vi "关键参数交互.vi"(9 "量程下拉列表":refnum<vi>, 10 "测量模式下拉列表":refnum<vi>, 11 "参数下拉列表":refnum<vi>) -> ()   [LabVIEW 2016]
uses:
  <vilib>/regexp/Match Regular Expression.xnode
panel:
  out "x != y?":T1
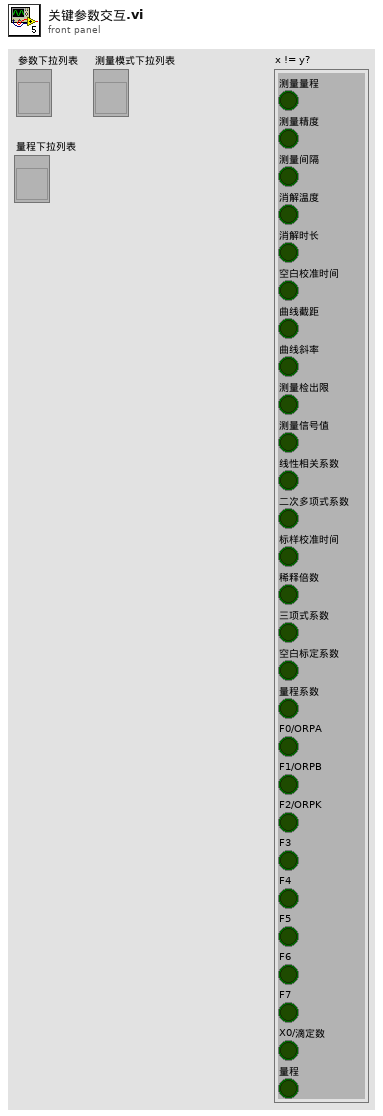
[diagram p1: front panel]
types:
  T1 = cluster{"测量量程":bool, "测量精度":bool, "测量间隔":bool, "消解温度":bool, "消解时长":bool, "空白校准时间":bool, "曲线截距":bool, "曲线斜率":bool, "测量检出限":bool, "测量信号值":bool, "线性相关系数":bool, "二次多项式系数":bool, "标样校准时间":bool, "稀释倍数":bool, "三项式系数":bool, "空白标定系数":bool, "量程系数":bool, "F0/ORPA":bool, "F1/ORPB":bool, "F2/ORPK":bool, "F3":bool, "F4":bool, "F5":bool, "F6":bool, "F7":bool, "X0/滴定数":bool, "量程":bool}
  T2 = cluster{"chose":string, "公式":cluster{"X^2":dbl, "X":dbl, "b":dbl}}
  T3 = cluster{"测量量程":dbl, "测量精度":dbl, "测量间隔":dbl, "消解温度":dbl, "消解时长":dbl, "空白校准时间":timestamp, "曲线截距":dbl, "曲线斜率":dbl, "测量检出限":dbl, "测量信号值":dbl, "线性相关系数":dbl, "二次多项式系数":dbl, "标样校准时间":timestamp, "稀释倍数":dbl, "三项式系数":dbl, "空白标定系数":dbl, "量程系数":dbl, "F0/ORPA":dbl, "F1/ORPB":dbl, "F2/ORPK":dbl, "F3":dbl, "F4":dbl, "F5":dbl, "F6":dbl, "F7":dbl, "X0/滴定数":dbl, "量程":dbl}
  T4 = cluster{"时间标识":timestamp, "设备":string, "日志信息":string, "流程参数":string}
  T5 = enum16{"", "水样测量", "标样核查", "零点核查", "跨度核查", "空白测试", "平行样测试", "加标回收"}
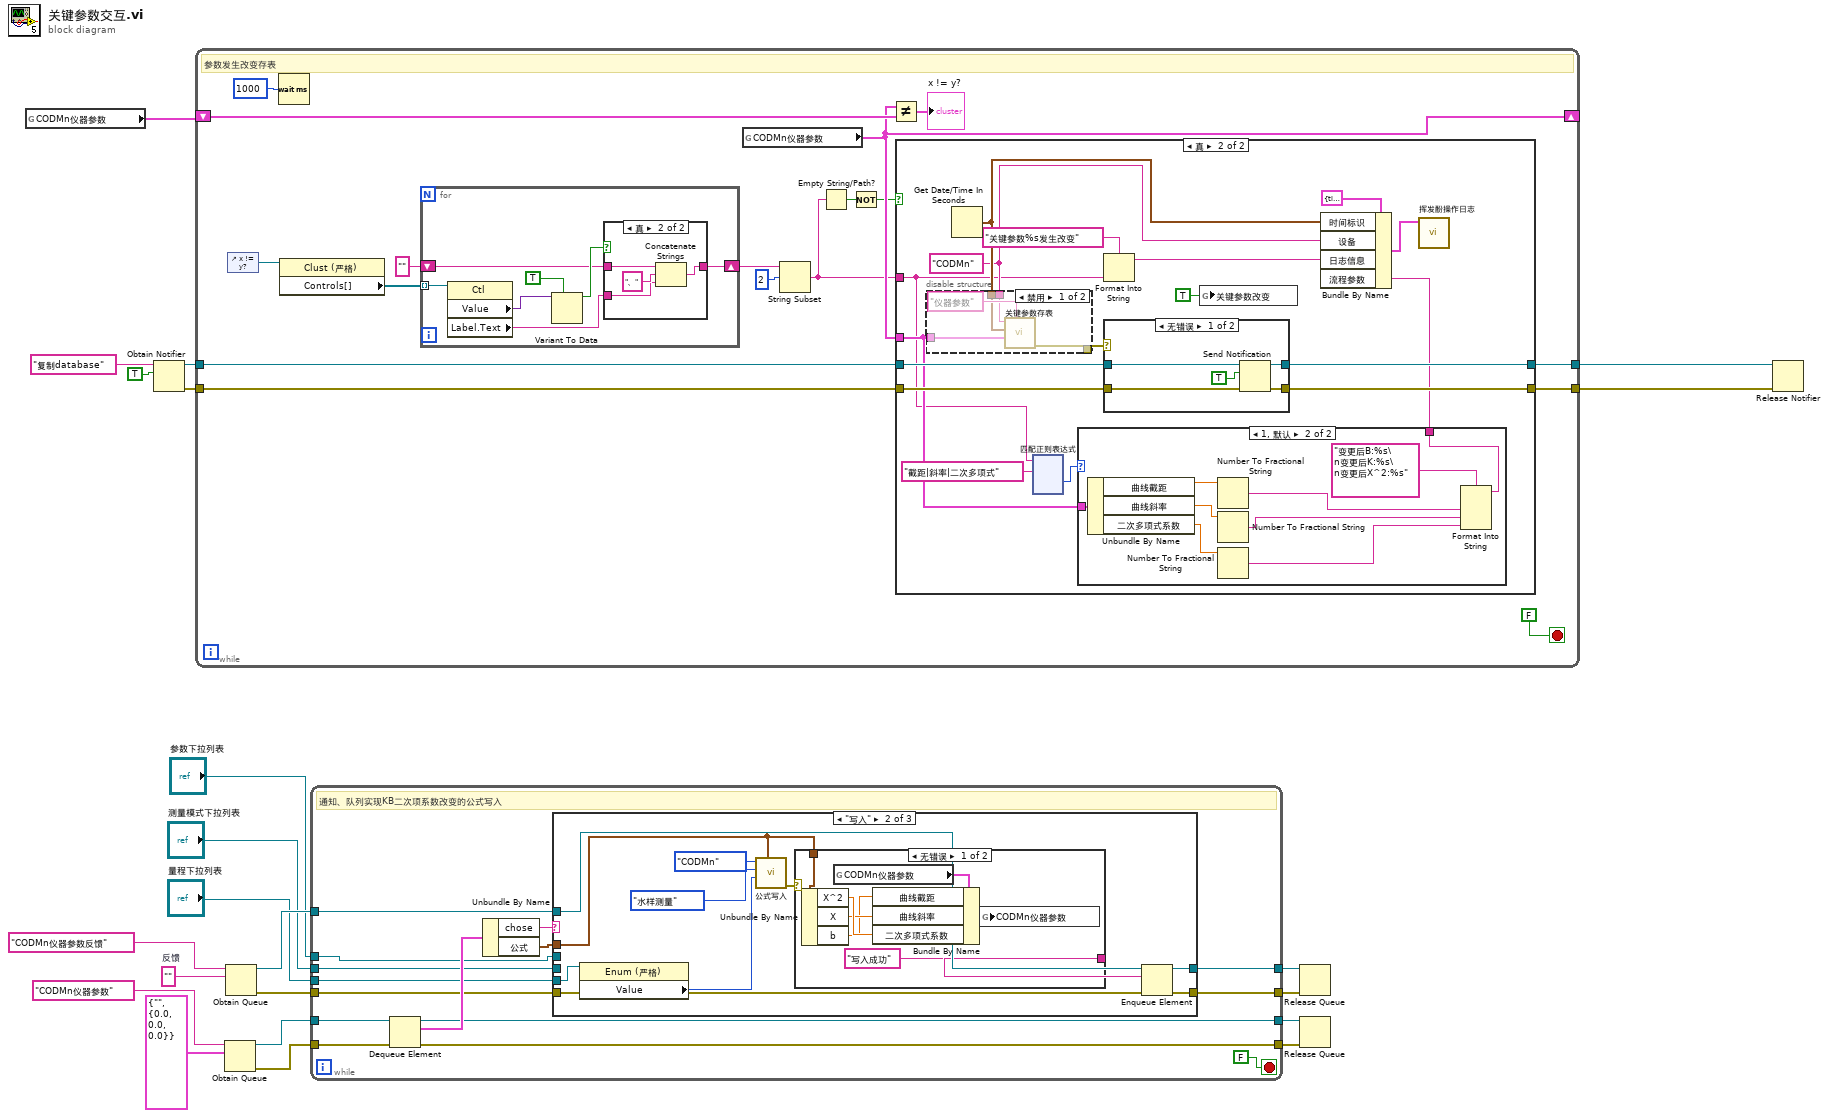
[diagram p0: block diagram]
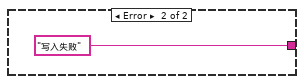
[diagram p3: hidden frame]
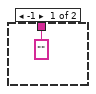
[diagram p8: hidden frame]
diagram:
  w15 = ""  # 反馈
  n1 = global read "挥发酚断电保存全局变量.vi" "CODMn仪器参数"() -> (w22:T3)
  n2 = Obtain Notifier(name (unnamed)="复制database" ("名称（未命名）"), notification data type=TRUE) -> (notifier out=w5:refnum<notifier>, error out=w4:errorcluster)  [unwired: 2 in, 1 out]
  n3 = while {
    shift-right: [w34] -> _
    shift-left: w22 -> [w37]
    tunnel: w5 -> [w33]
    tunnel: w4 -> [w32]
    tunnel: [w31] -> w3
    tunnel: [w30] -> w2
    stop <- FALSE stop-if-true
    # "参数发生改变存表"
    n4 = control-ref of="x != y?"() -> (w35:refnum<vi>)
    n5 = Wait (ms)(milliseconds to wait=u32 1000 ("等待时间（毫秒）")) -> ()  [unwired: 1 out]
    n6 = property class="Clust (严格)"(reference=w35) -> ("Controls[]"=w26:refnum<vi>[])  [unwired: 1 in, 2 out]
    n7 = for {
      tunnel: w26 -> [w46] mode=indexing
      shift-right: [w40] -> w28
      shift-left: "" -> [w42]
      n8 = property class="Ctl"(reference=w46) -> ("Value"=w44:variant, "Label.Text"=w41:string)  [unwired: 1 in, 2 out]
      n9 = Variant To Data(type=TRUE, Variant=w44) -> (data=w43:bool)  [unwired: 1 in, 1 out]
      n10 = case shown="真" w43 {
        tunnel: w42 -> [w47 w51]
        tunnel: w41 -> [_ w48]
        tunnel: [w47 w50] -> w40
        frame False {
        }
        frame True {
          n11 = Concatenate Strings(w51, "、", w48) -> (w50:string)
        }
      }
    }
    n12 = global read "挥发酚断电保存全局变量.vi" "CODMn仪器参数"() -> (w34:T3)
    n13 = String Subset(string=w28, offset (0)=2 ("偏移量(0)")) -> (substring=w23:string)  [unwired: 1 in]
    n14 = Empty String/Path?(string/path=w23) -> (empty?=w25:bool)
    n15 = Not(x=w25) -> (.not. x?=w24:bool)
    n16 = Not Equal?(x=w34, y=w37) -> (x != y?=→"x != y?":T1)
    n17 = case shown="真" w24 {
      tunnel: w34 -> [_ w59]
      tunnel: w23 -> [_ w56]
      tunnel: w33 -> [w53 w64]
      tunnel: w32 -> [w52 w63]
      tunnel: [w53 w61] -> w31
      tunnel: [w52 w60] -> w30
      frame False {
      }
      frame True {
        w67 = "CODMn" ("仪器名称")
        n18 = Get Date/Time In Seconds() -> (seconds since 1Jan1904=w68:timestamp)
        n19 = disable-structure shown="禁用" {
          disable-tunnel: w68 -> [w74 _]
          disable-tunnel: w67 -> [w73 _]
          disable-tunnel: [w72 _] -> w62
          disable-tunnel: w59 -> [w71 _]
          frame Disabled {
            n20 = call "关键参数存表.vi"("table"="仪器参数", "仪器参数"=w71, "datatime"=w74, "仪器名称"=w73) -> ("error out"=w72:errorcluster)  [unwired: 7 in]
          }
          frame Enabled {
          }
        }
        n21 = xnode "匹配正则表达式"("输入字符串"=w56, "正则表达式"="截距|斜率|二次多项式") -> ("匹配后偏移量"=w55:i32)  [unwired: 4 in, 4 out]
        n22 = case shown="1, 默认" w55 {
          tunnel: w59 -> [_ w198]
          tunnel: ["" w191] -> w58
          frame -1 {
          }
          frame 1, Default {
            n23 = Unbundle By Name(w198) -> ("曲线截距"=w197:dbl, "曲线斜率"=w196:dbl, "二次多项式系数"=w195:dbl)
            n24 = Number To Fractional String(number=w197) -> (F-format string=w194:string)  [unwired: 3 in]
            n25 = Number To Fractional String(number=w196) -> (F-format string=w193:string)  [unwired: 3 in]
            n26 = Number To Fractional String(number=w195) -> (F-format string=w192:string)  [unwired: 3 in]
            n27 = Format Into String(format string="变更后B:%s\n变更后K:%s\n变更后X^2:%s" ("格式字符串"), w194, w193, w192) -> (resulting string=w191:string)  [unwired: 2 in, 1 out]
          }
        }
        n28 = Format Into String(format string="关键参数%s发生改变" ("格式字符串"), w56) -> (resulting string=w65:string)  [unwired: 2 in, 1 out]
        n29 = case shown="无错误" w62 {
          tunnel: w64 -> [w204 w206]
          tunnel: w63 -> [w203 w205]
          tunnel: [w201 w206] -> w61
          tunnel: [w200 w205] -> w60
          frame No Error {
            n30 = Send Notification(notification=TRUE ("通知"), notifier=w204, error in (no error)=w203) -> (notifier out=w201:refnum<notifier>, error out=w200:errorcluster)
          }
          frame Error {
          }
        }
        n31 = global write "挥发酚断电保存全局变量.vi" "关键参数改变"(TRUE ("关键参数改变")) -> ()
        n32 = Bundle By Name(cluster=T4 {"时间标识"=timestamp(0 s since 1904-01-01), "设备"="", "日志信息"="", "流程参数"=""} ("data in"), "时间标识"=w68, "设备"=w67, "日志信息"=w65, "流程参数"=w58) -> (w69:T4)
        n33 = call "挥发酚操作日志.vi"("data in"=w69) -> ()  [unwired: 11 in]
      }
    }
  }
  n34 = Obtain Queue(name (unnamed)="CODMn仪器参数" ("名称（未命名）"), element data type=T2 {"chose"="", "公式"={"X^2"=0.0, "X"=0.0, "b"=0.0}}) -> (queue out=w11:refnum<queue>, error out=w10:errorcluster)  [unwired: 3 in, 1 out]
  n35 = Obtain Queue(name (unnamed)="CODMn仪器参数反馈" ("名称（未命名）"), element data type=w15) -> (queue out=w16:refnum<queue>, error out=w14:errorcluster)  [unwired: 3 in, 1 out]
  n36 = while {
    tunnel: w11 -> [w220]
    tunnel: w10 -> [w219]
    tunnel: [w211] -> w19
    tunnel: [w210] -> w18
    tunnel: w16 -> [w215]
    tunnel: w14 -> [w214]
    tunnel: [w213] -> w13
    tunnel: [w212] -> w12
    tunnel: "参数下拉列表" -> [w209]
    tunnel: "测量模式下拉列表" -> [w208]
    tunnel: "量程下拉列表" -> [w207]
    stop <- FALSE stop-if-true
    # "通知、队列实现KB二次项系数改变的公式写入"
    n37 = Dequeue Element(queue=w220, error in (no error)=w219) -> (queue out=w211:refnum<queue>, element=w218:T2, error out=w210:errorcluster)  [unwired: 1 in, 1 out]
    n38 = Unbundle By Name(w218) -> ("chose"=w217:string, "公式"=w216:cluster{"X^2":dbl, "X":dbl, "b":dbl})
    n39 = case shown="\"写入\"" w217 {
      tunnel: w216 -> [_ w228 _]
      tunnel: w215 -> [w223 w233 w244]
      tunnel: w214 -> [w222 w231 w243]
      tunnel: [w223 w230 w244] -> w213
      tunnel: [w222 w229 w243] -> w212
      tunnel: w209 -> [_ _ _]
      tunnel: w208 -> [_ _ _]
      tunnel: w207 -> [_ w225 _]
      frame "假", Default {
      }
      frame "写入" {
        n40 = property class="Enum (严格)"(reference=w225) -> ("Value"=w224:enum16{"低量程1", "低量程2", "高量程1", "高量程2"})  [unwired: 1 in, 2 out]
        n41 = call "公式写入.vi"("公式"=w228, "量程"=w224, "测量模式"=T5."水样测量", "测量参数"=enum16{"CODMn"}."CODMn") -> ("error out"=w234:errorcluster)  [unwired: 7 in]
        n42 = case shown="无错误" w234 {
          tunnel: ["写入成功" ("消息") "写入失败" ("消息")] -> w232
          tunnel: w228 -> [w238 _]
          frame No Error {
            n43 = Unbundle By Name(w238) -> ("X^2"=w237:dbl, "X"=w236:dbl, "b"=w235:dbl)
            n44 = global read "挥发酚断电保存全局变量.vi" "CODMn仪器参数"() -> (w239:T3)
            n45 = Bundle By Name(cluster=w239, "曲线截距"=w235, "曲线斜率"=w236, "二次多项式系数"=w237) -> (w240:T3)
            n46 = global write "挥发酚断电保存全局变量.vi" "CODMn仪器参数"(w240) -> ()
          }
          frame Error {
          }
        }
        n47 = Enqueue Element(queue=w233, element=w232, error in (no error)=w231) -> (queue out=w230:refnum<queue>, error out=w229:errorcluster)  [unwired: 1 in, 1 out]
      }
      frame "读取" {
      }
    }
  }
  n48 = Release Queue(queue=w13, error in (no error)=w12) -> ()  [unwired: 1 in, 3 out]
  n49 = Release Queue(queue=w19, error in (no error)=w18) -> ()  [unwired: 1 in, 3 out]
  n50 = Release Notifier(notifier=w3, error in (no error)=w2) -> ()  [unwired: 1 in, 3 out]
